vi "Generate Sine.vi"(4 "错误输入":cluster{"状态":bool, "代码":i32, "源":string}, 5 "数值":i32) -> (0 "错误输出":cluster{"状态":bool, "代码":i32, "源":string}, 2 "正弦波":dbl)   [LabVIEW 2012]
doc: "该VI逐点生成正弦波。"
uses:
  <vilib>/ptbypt/NI_PtbyPt.lvlib
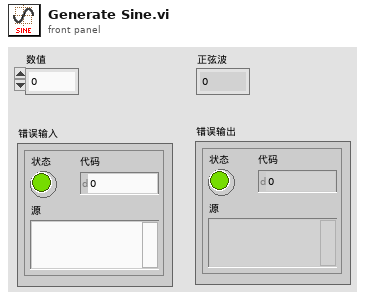
[diagram p1: front panel]
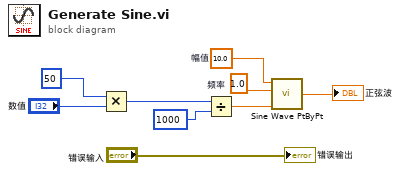
[diagram p0: block diagram]
diagram:
  w4 = 1.0  # 频率
  w3 = 10.0  # 幅值
  n1 = Multiply ("乘")(x=u32 50 ("等待时间（毫秒）"), y="数值") -> (x*y=w8:u32)
  n2 = Divide ("除")(x=w8, y=u32 1000) -> (x/y=w9:dbl)
  n3 = call <vilib>:"Sine Wave PtByPt.vi"("time"=w9, "frequency"=w4, "amplitude"=w3) -> ("sine wave"=→"正弦波":dbl)  [unwired: 1 in]
  "错误输出" <- "错误输入"
